vi "Flush.vi"(8 "error in":errorcluster, 11 "CanHandleIn":T1) -> (0 "error out":errorcluster, 3 "CanHandleOut":T1)   [LabVIEW 2011, in "Konvolucio MCAN120803.lvlib"]
uses:
  <instrlib>/Konvolucio MCAN120803/Konvolucio MCAN120803.lvlib
  <instrlib>/Konvolucio MCAN120803/Types/CanHandleType.ctl
  C:/Program Files/National Instruments/LabVIEW 2011/instr.lib/Konvolucio MCAN120803/Private/Konvolucio.MCAN120803.API.dll
  Private/Konvolucio.MCAN120803.API.dll
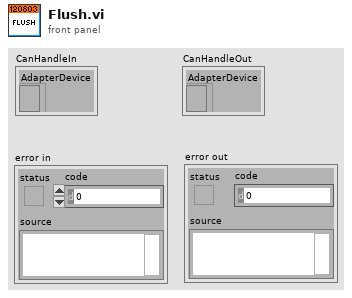
[diagram p1: front panel]
types:
  T1 = typedef "Konvolucio MCAN120803.lvlib/CanHandleType.ctl" = cluster{"AdapterDevice":refnum<k24>}
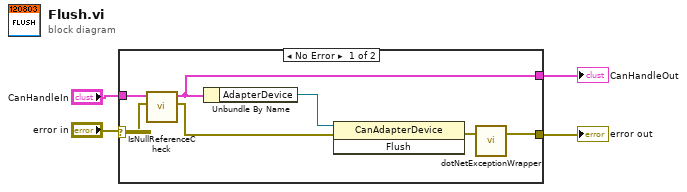
[diagram p0: block diagram]
diagram:
  n1 = case shown="No Error" "error in" {
    selector: "error in" -> [w5 w13]
    tunnel: [w10 w13] -> w4
    tunnel: "CanHandleIn" -> [w7 w12]
    tunnel: [w8 w12] -> w1
    frame No Error {
      n2 = call <instrlib>:"IsNullReferenceCheck.vi"("error in"=w5, "MCanHandleIn"=w7) -> ("error out"=w6:errorcluster, "MCanHandleOut"=w8:T1)  [unwired: 5 in]
      n3 = Unbundle By Name(w8) -> ("AdapterDevice"=w11:refnum<k24>)
      n4 = invoke class="CanAdapterDevice" method="Flush"(reference=w11, error in=w6) -> (error out=w9:errorcluster)  [unwired: 1 in, 2 out]
      n5 = call <instrlib>:"dotNetExceptionWrapper.vi"("error in"=w9) -> ("error out"=w10:errorcluster)  [unwired: 2 in]
    }
    frame Error {
    }
  }
  "error out" <- w4
  "CanHandleOut" <- w1
